vi "Parse Text Message.vi"(9 "Characters Per Line":i32=1 min=1, 11 "Input String":string) -> (1 "Number Of Lines":i32=12, 3 "Output String":string="\r\n")   [LabVIEW 2019, in "ErrorHandler.lvclass"]
doc: "Developed by Kevin Thompson\nkevin@thompsonengineering.net\n\nCopyright 2018\nThompson Engineering, LLC"
uses:
  ErrorHandler.lvclass
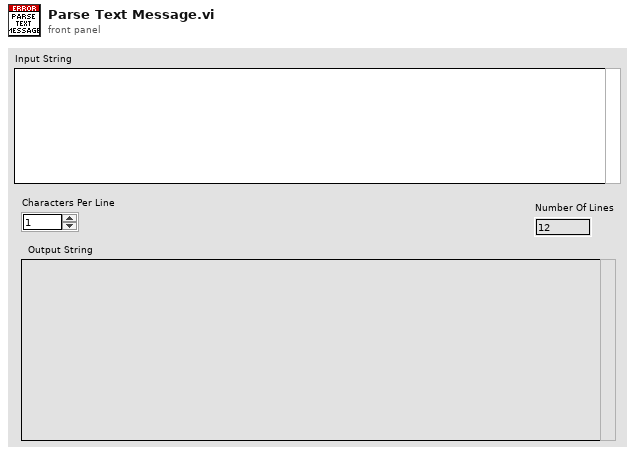
[diagram p1: front panel]
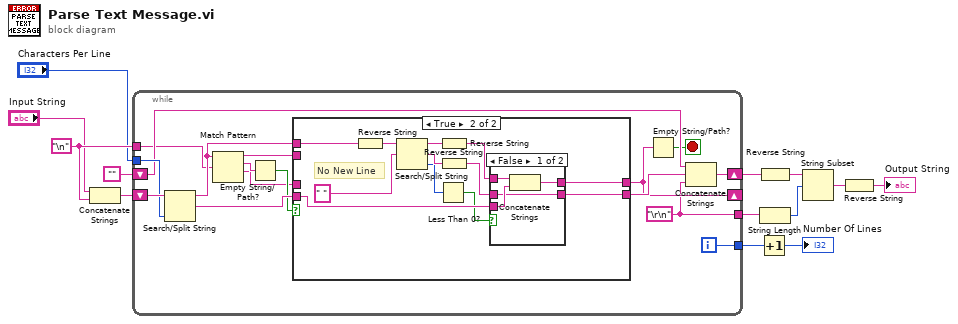
[diagram p0: block diagram]
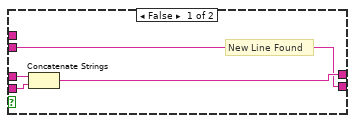
[diagram p2: hidden frame]
diagram:
  w13 = "\n"
  n1 = Concatenate Strings("Input String", w13) -> (w5:string)
  n2 = while {
    tunnel: [w21] -> w3
    tunnel: "Characters Per Line" -> [w26]
    shift-left: "" -> [w22]
    shift-right: [w24] -> w12
    shift-left: w5 -> [w28]
    shift-right: [w17] -> _
    tunnel: w13 -> [w15]
    tunnel: [w14] -> w7
    i -> [w21]
    stop <- w16 stop-if-true
    w14 = "\r\n"
    n3 = Search/Split String(string=w28, offset (0)=w26) -> (substring before match=w20:string, match + rest of string=w27:string)  [unwired: 1 in, 1 out]
    n4 = Match Pattern(string=w20, regular expression=w15) -> (before substring=w25:string, match substring=w29:string, after substring=w18:string)  [unwired: 1 in, 1 out]
    n5 = Empty String/Path?(string/path=w29) -> (empty?=w19:bool)
    n6 = case shown="True" w19 {
      tunnel: w20 -> [_ w45]
      tunnel: w27 -> [w32 w38]
      tunnel: [w31 w37] -> w17
      tunnel: w25 -> [w30 _]
      tunnel: w18 -> [w33 _]
      tunnel: [w30 w35] -> w23
      frame False {
        # "New Line Found"
        n7 = Concatenate Strings(w33, w32) -> (w31:string)
      }
      frame True {
        # "No New Line"
        n8 = Reverse String(1:w45) -> (0:w44:string)
        n9 = Search/Split String(string=w44, search string/char (-)=" ") -> (substring before match=w42:string, match + rest of string=w41:string, offset of match=w40:i32)  [unwired: 1 in]
        n10 = Less Than 0?(x=w40) -> (x < 0?=w34:bool)
        n11 = Reverse String(1:w42) -> (0:w39:string)
        n12 = Reverse String(1:w41) -> (0:w36:string)
        n13 = case shown="False" w34 {
          tunnel: w39 -> [w49 w50]
          tunnel: [w48 w51] -> w37
          tunnel: w38 -> [w47 w51]
          tunnel: w36 -> [w46 _]
          tunnel: [w46 w50] -> w35
          frame False {
            n14 = Concatenate Strings(w49, w47) -> (w48:string)
          }
          frame True {
          }
        }
      }
    }
    n15 = Empty String/Path?(string/path=w17) -> (empty?=w16:bool)
    n16 = Concatenate Strings(w22, w23, w14) -> (w24:string)
  }
  n17 = Increment(x=w3) -> (x+1=→"Number Of Lines":i32)
  n18 = Reverse String(1:w12) -> (0:w9:string)
  n19 = String Length(string=w7) -> (length=w8:i32)
  n20 = String Subset(string=w9, offset (0)=w8) -> (substring=w10:string)  [unwired: 1 in]
  n21 = Reverse String(1:w10) -> (0:→"Output String":string)
